vi "GlobalArmPosition.vi"() -> ()   [LabVIEW 2014]
panel:
  in  "Right Arm Home Voltage":dbl
  in  "Left Arm Home Voltage":dbl
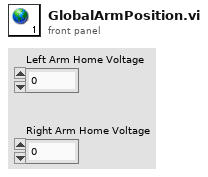
[diagram p1: front panel]
diagram:
